vi "Practica4_serieLed.vi"() -> ()   [LabVIEW 2015]
uses:
  <vilib>/LabVIEW Interface for Arduino/Type Defs/Pin Mode.ctl
  <vilib>/LabVIEW Interface for Arduino/LabVIEW Interface for Arduino.lvlib
panel:
  in  "stop":bool
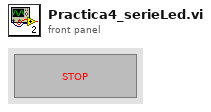
[diagram p1: front panel]
types:
  T1 = typedef "LabVIEW Interface for Arduino.lvlib/Pin Mode.ctl" = enum8{"Input", "Output"}
  T2 = typedef "LabVIEW Interface for Arduino.lvlib/Arduino Resource.ctl" = cluster{"VISA resource":refnum<visa-resource-name>, "Board Type":T3, "Connection Type":enum8{"USB / Serial"}, "Bytes Per Packet (15)":u8}
  T3 = typedef "LabVIEW Interface for Arduino.lvlib/Board Type.ctl" = enum16{"Uno", "Dimuelanove w/Atmega 328", "Mega 2560"}
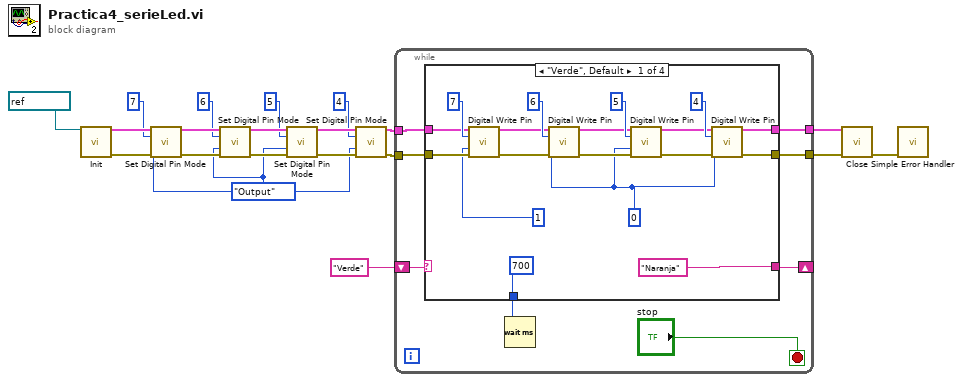
[diagram p0: block diagram]
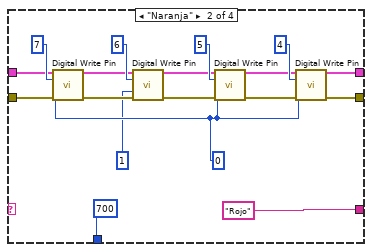
[diagram p2: hidden frame]
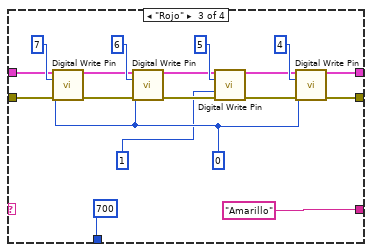
[diagram p3: hidden frame]
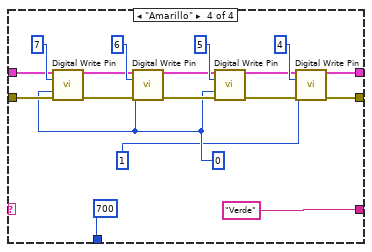
[diagram p4: hidden frame]
diagram:
  w10 = Pin_Mode."Output" ("Pin Mode (Input)")
  n1 = call <vilib>:"Init.vi"("VISA resource"=refnum<visa-resource-name> "COM3") -> ("Arduino Resource"=w20:T2, "error out"=w19:errorcluster)  [unwired: 17 in]
  n2 = call <vilib>:"Set Digital Pin Mode.vi"("Arduino Resource"=w20, "Digital I/O Pin"=u8 7, "Pin Mode (Input)"=w10, "error in"=w19) -> ("Arduino Resource"=w17:T2, "error out"=w12:errorcluster)  [unwired: 10 in]
  n3 = call <vilib>:"Set Digital Pin Mode.vi"("Arduino Resource"=w17, "Digital I/O Pin"=u8 6, "Pin Mode (Input)"=w10, "error in"=w12) -> ("Arduino Resource"=w16:T2, "error out"=w13:errorcluster)  [unwired: 10 in]
  n4 = call <vilib>:"Set Digital Pin Mode.vi"("Arduino Resource"=w16, "Digital I/O Pin"=u8 5, "Pin Mode (Input)"=w10, "error in"=w13) -> ("Arduino Resource"=w15:T2, "error out"=w14:errorcluster)  [unwired: 10 in]
  n5 = call <vilib>:"Set Digital Pin Mode.vi"("Arduino Resource"=w15, "Digital I/O Pin"=u8 4, "Pin Mode (Input)"=w10, "error in"=w14) -> ("Arduino Resource"=w6:T2, "error out"=w5:errorcluster)  [unwired: 10 in]
  n6 = while {
    tunnel: w6 -> [w25]
    tunnel: w5 -> [w24]
    shift-right: [w27] -> _
    shift-left: "Verde" -> [w26]
    tunnel: [w22] -> w3
    tunnel: [w21] -> w2
    stop <- "stop" stop-if-true
    n7 = case shown="\"Verde\", Default" w26 {
      tunnel: ["Naranja" "Rojo" "Amarillo" "Verde"] -> w27
      tunnel: w25 -> [w35 w53 w71 w89]
      tunnel: w24 -> [w34 w52 w70 w88]
      tunnel: [u32 700 ("milliseconds to wait") u32 700 ("milliseconds to wait") u32 700 ("milliseconds to wait") u32 700 ("milliseconds to wait")] -> w23
      tunnel: [w30 w48 w66 w84] -> w22
      tunnel: [w29 w47 w65 w83] -> w21
      frame "Verde", Default {
        w31 = u8 0 ("Value (0)")
        n8 = call <vilib>:"Digital Write Pin.vi"("Arduino Resource"=w35, "Digital I/O Pin (0)"=u8 7, "Value (0)"=u8 1, "error in"=w34) -> ("Arduino Resource"=w37:T2, "error out"=w40:errorcluster)  [unwired: 10 in]
        n9 = call <vilib>:"Digital Write Pin.vi"("Arduino Resource"=w37, "Digital I/O Pin (0)"=u8 6, "Value (0)"=w31, "error in"=w40) -> ("Arduino Resource"=w38:T2, "error out"=w41:errorcluster)  [unwired: 10 in]
        n10 = call <vilib>:"Digital Write Pin.vi"("Arduino Resource"=w38, "Digital I/O Pin (0)"=u8 5, "Value (0)"=w31, "error in"=w41) -> ("Arduino Resource"=w39:T2, "error out"=w42:errorcluster)  [unwired: 10 in]
        n11 = call <vilib>:"Digital Write Pin.vi"("Arduino Resource"=w39, "Digital I/O Pin (0)"=u8 4, "Value (0)"=w31, "error in"=w42) -> ("Arduino Resource"=w30:T2, "error out"=w29:errorcluster)  [unwired: 10 in]
      }
      frame "Naranja" {
        w50 = u8 0 ("Value (0)")
        n12 = call <vilib>:"Digital Write Pin.vi"("Arduino Resource"=w53, "Digital I/O Pin (0)"=u8 7, "Value (0)"=w50, "error in"=w52) -> ("Arduino Resource"=w55:T2, "error out"=w58:errorcluster)  [unwired: 10 in]
        n13 = call <vilib>:"Digital Write Pin.vi"("Arduino Resource"=w55, "Digital I/O Pin (0)"=u8 6, "Value (0)"=u8 1, "error in"=w58) -> ("Arduino Resource"=w56:T2, "error out"=w59:errorcluster)  [unwired: 10 in]
        n14 = call <vilib>:"Digital Write Pin.vi"("Arduino Resource"=w56, "Digital I/O Pin (0)"=u8 5, "Value (0)"=w50, "error in"=w59) -> ("Arduino Resource"=w57:T2, "error out"=w60:errorcluster)  [unwired: 10 in]
        n15 = call <vilib>:"Digital Write Pin.vi"("Arduino Resource"=w57, "Digital I/O Pin (0)"=u8 4, "Value (0)"=w50, "error in"=w60) -> ("Arduino Resource"=w48:T2, "error out"=w47:errorcluster)  [unwired: 10 in]
      }
      frame "Rojo" {
        w68 = u8 0 ("Value (0)")
        n16 = call <vilib>:"Digital Write Pin.vi"("Arduino Resource"=w71, "Digital I/O Pin (0)"=u8 7, "Value (0)"=w68, "error in"=w70) -> ("Arduino Resource"=w73:T2, "error out"=w76:errorcluster)  [unwired: 10 in]
        n17 = call <vilib>:"Digital Write Pin.vi"("Arduino Resource"=w73, "Digital I/O Pin (0)"=u8 6, "Value (0)"=w68, "error in"=w76) -> ("Arduino Resource"=w74:T2, "error out"=w77:errorcluster)  [unwired: 10 in]
        n18 = call <vilib>:"Digital Write Pin.vi"("Arduino Resource"=w74, "Digital I/O Pin (0)"=u8 5, "Value (0)"=u8 1, "error in"=w77) -> ("Arduino Resource"=w75:T2, "error out"=w78:errorcluster)  [unwired: 10 in]
        n19 = call <vilib>:"Digital Write Pin.vi"("Arduino Resource"=w75, "Digital I/O Pin (0)"=u8 4, "Value (0)"=w68, "error in"=w78) -> ("Arduino Resource"=w66:T2, "error out"=w65:errorcluster)  [unwired: 10 in]
      }
      frame "Amarillo" {
        w86 = u8 0 ("Value (0)")
        n20 = call <vilib>:"Digital Write Pin.vi"("Arduino Resource"=w89, "Digital I/O Pin (0)"=u8 7, "Value (0)"=w86, "error in"=w88) -> ("Arduino Resource"=w91:T2, "error out"=w94:errorcluster)  [unwired: 10 in]
        n21 = call <vilib>:"Digital Write Pin.vi"("Arduino Resource"=w91, "Digital I/O Pin (0)"=u8 6, "Value (0)"=w86, "error in"=w94) -> ("Arduino Resource"=w92:T2, "error out"=w95:errorcluster)  [unwired: 10 in]
        n22 = call <vilib>:"Digital Write Pin.vi"("Arduino Resource"=w92, "Digital I/O Pin (0)"=u8 5, "Value (0)"=w86, "error in"=w95) -> ("Arduino Resource"=w93:T2, "error out"=w96:errorcluster)  [unwired: 10 in]
        n23 = call <vilib>:"Digital Write Pin.vi"("Arduino Resource"=w93, "Digital I/O Pin (0)"=u8 4, "Value (0)"=u8 1, "error in"=w96) -> ("Arduino Resource"=w84:T2, "error out"=w83:errorcluster)  [unwired: 10 in]
      }
    }
    n24 = Wait (ms)(milliseconds to wait=w23) -> ()  [unwired: 1 out]
  }
  n25 = call <vilib>:"Close.vi"("Arduino Resource"=w3, "error in"=w2) -> ("error out"=w1:errorcluster)  [unwired: 13 in]
  n26 = call <vilib>:"Simple Error Handler.vi"("error in (no error)"=w1) -> ()  [unwired: 4 in, 5 out]
